vi "Actual Sample Rate.vi"(8 "error in (no error)":errorcluster {"code" format="%.0x"}, 11 "VISA Resource Name":refnum<visa-resource-name>) -> (0 "error out":errorcluster {"code" format="%.0x"}, 2 "sample rate":dbl caption="Sample Rate" format="%^.2e", 3 "VISA Resource Name Out":refnum<visa-resource-name>)   [LabVIEW 2011, in "Agilent 546XX Series.lvlib"]
doc: "This VI returns the effective sample rate of the acquired waveform using the current configuration in samples per second."
uses:
  Agilent 546XX Series.lvlib
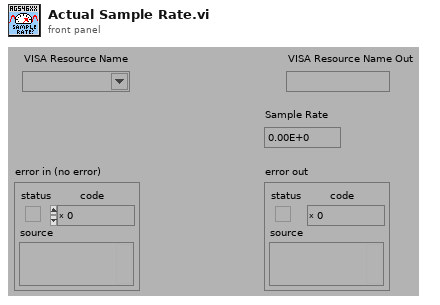
[diagram p1: front panel]
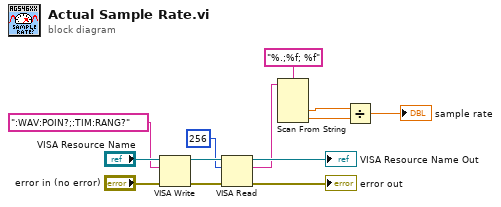
[diagram p0: block diagram]
diagram:
  n1 = VISA Write(VISA resource name="VISA Resource Name", write buffer=":WAV:POIN?;:TIM:RANG?", error in (no error)="error in (no error)") -> (VISA resource name out=w9:refnum<visa-resource-name>, error out=w8:errorcluster)  [unwired: 1 out]
  n2 = VISA Read(VISA resource name=w9, byte count=u32 256, error in (no error)=w8) -> (VISA resource name out=→"VISA Resource Name Out":refnum<visa-resource-name>, read buffer=w5:string, error out=→"error out":errorcluster)  [unwired: 1 out]
  n3 = Scan From String(format string="%.;%f; %f", input string=w5) -> (output 1=w3:dbl, output 2=w2:dbl)  [unwired: 4 in, 3 out]
  n4 = Divide(x=w3, y=w2) -> (x/y=→"sample rate":dbl)
